vi "Write prev s4 acq config.vi"(8 "error in (no error)":errorcluster, 9 "prev SET parameters":cluster{"suffix":string, "#CYCLES":u32}={"suffix"="", "#CYCLES"=1}, 10 "prev s4 acq config":T1={"#SEQS"=1, "WAVEPLATE_POS"=0, "Waveplate positions"=[]}, 11 "SPARC4_Channel in":refnum<class "SPARC4_Channel.lvclass">) -> (0 "error out":errorcluster, 3 "SPARC4_Channel out":refnum<class "SPARC4_Channel.lvclass">)   [LabVIEW 2018, in "SPARC4_Channel.lvclass"]
uses:
  SPARC4_Channel.lvclass
  SPARC4_Channel.lvclass/SPARC4_Channel.ctl
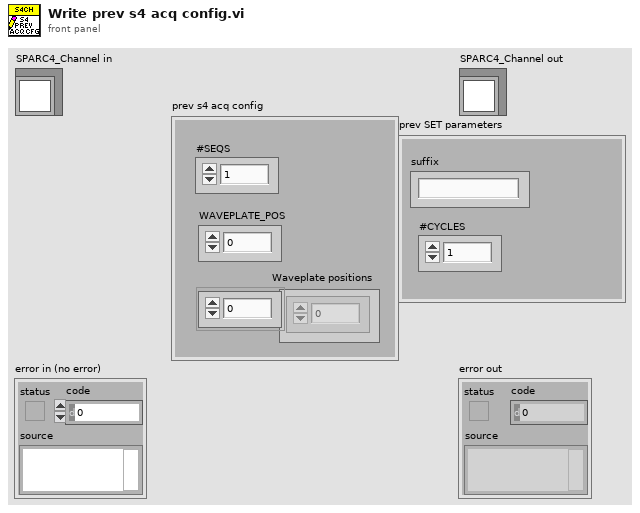
[diagram p1: front panel]
types:
  T1 = cluster{"#SEQS":u32, "WAVEPLATE_POS":u16, "Waveplate positions":u8[]}
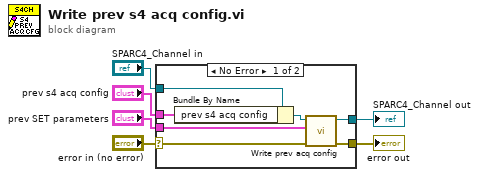
[diagram p0: block diagram]
diagram:
  n1 = case shown="No Error" "error in (no error)" {
    selector: "error in (no error)" -> [w8 w14]
    tunnel: [w9 w14] -> w5
    tunnel: [w10 w15] -> w3
    tunnel: "SPARC4_Channel in" -> [w13 w15]
    tunnel: "prev s4 acq config" -> [w12 _]
    tunnel: "prev SET parameters" -> [w7 _]
    frame No Error {
      n2 = Bundle By Name(cluster=w13, "prev s4 acq config"=w12) -> (w11:refnum<class "SPARC4_Channel.lvclass">)
      n3 = call-dynamic "Write prev acq config.vi"("error in (no error)"=w8, "prev SET parameters"=w7, "Channel in"=w11) -> ("error out"=w9:errorcluster, "Channel out"=w10:refnum<class "SPARC4_Channel.lvclass">)  [unwired: 7 in]
    }
    frame Error {
    }
  }
  "error out" <- w5
  "SPARC4_Channel out" <- w3
